vi "greaterNum.vi"() -> ()   [LabVIEW 2019]
panel:
  out "Average":dbl
  out "min value":dbl
  out "max value":dbl
  in  "Array":dbl[](array[numeric])
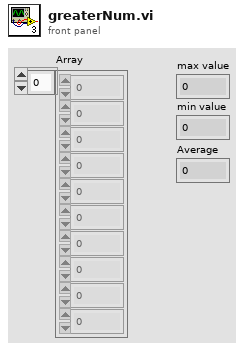
[diagram p1: front panel]
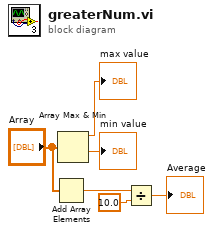
[diagram p0: block diagram]
diagram:
  n1 = Add Array Elements(numeric array="Array") -> (sum=w3:dbl)
  n2 = Array Max & Min(array="Array") -> (max value=→"max value":dbl, min value=→"min value":dbl)  [unwired: 2 out]
  n3 = Divide(x=w3, y=10.0) -> (x/y=→"Average":dbl)
